vi "Start.vi"(6 "Teller":T1 {"AbsoluteTime" format="%<%x %.3X>T"}, 8 "Error in":errorcluster, 11 "Base Actor in":refnum<class "BaseActor.lvclass">) -> (0 "Error out":errorcluster, 3 "Base Actor out":refnum<class "BaseActor.lvclass">)   [LabVIEW 2020, in "jettl.lvlib" / "BaseActor.lvlib" / "BaseActor.lvclass"]
doc: "jettl 6.14.1.98\nNathan Davis - Nathan Davis\nCopyright (c) 2026, Nathan Davis\nMIT"
uses:
  BaseActor.lvclass
  MessageMetadata.ctl
  jettl.lvlib
  Lifetime.ctl
  TellOrigin.ctl
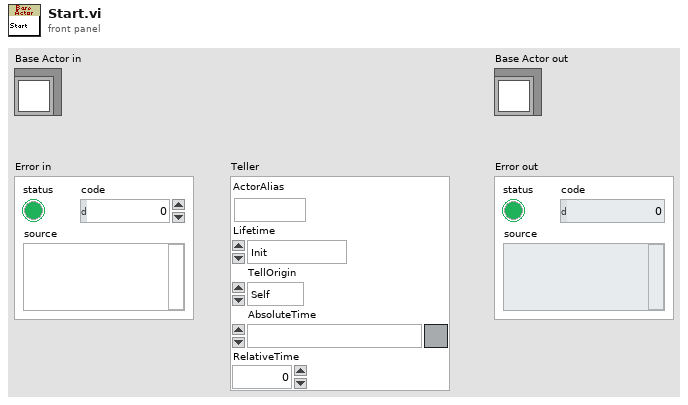
[diagram p1: front panel]
types:
  T1 = typedef "jettl.lvlib/MessageMetadata.ctl" = cluster{"ActorAlias":string, "Lifetime":T2, "TellOrigin":T3, "AbsoluteTime":timestamp, "RelativeTime":dbl}
  T2 = typedef "jettl.lvlib/Lifetime.ctl" = enum16{"Init", "Spawn", "Setup", "TeardownBeforeRunning", "Running", "StopCalled", "StoppingWithComponents", "StoppingNoComponents", "TeardownAfterRunning", "Stopped"}
  T3 = typedef "jettl.lvlib/TellOrigin.ctl" = enum16{"Self", "Mediator", "Component"}
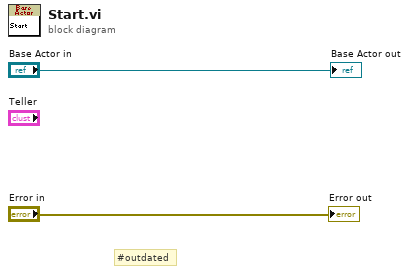
[diagram p0: block diagram]
diagram:
  # "#outdated"
  "Base Actor out" <- "Base Actor in"
  "Error out" <- "Error in"
